vi "Browse for XNET Database.vi"(8 "error in (no error)":errorcluster) -> (0 "error out":errorcluster, 1 "J1939 Monitor Settings":T1 {"Name" format="%.0x"}, 2 "Cancel Out":bool, 3 "J1939 XNET Settings":T2={"Database"="", "Cluster"="", "Port"="", "Baud rate [Bd]"=0, "Termination"=0, "Incoming Rate"=0, "Outcoming Rate"=0, "Write Decimation"=1} {"Termination" items=["Off", "On"]})   [LabVIEW 2015, in "J1939 Addon System Explorer.lvlib"]
uses:
  J1939 Addon System Explorer.lvlib
  Types/XNET Port.ctl
  Shared/Types/XNET Settings.ctl
  Shared/Types/Monitor Settings.ctl
  <resource>/objmgr/xnet.rc
  Shared/J1939 Addon Shared.lvlib
panel:
  in  "Name":u64=1
  in  "Address":u8
  in  "Baud rate [Bd]":u32=500000
  in  "Select CAN Cluster":u16(ring) items=["j1939.Cluster"]
  in  "XNET CAN Port":T3 items=["CAN 1", "CAN 2", "CAN 3", "CAN 4", "CAN 5", "CAN 6", "CAN 7", "CAN 8"]
  in  "Cancel":bool
  in  "Select":bool
  in  "XNET Database":refnum<k21>
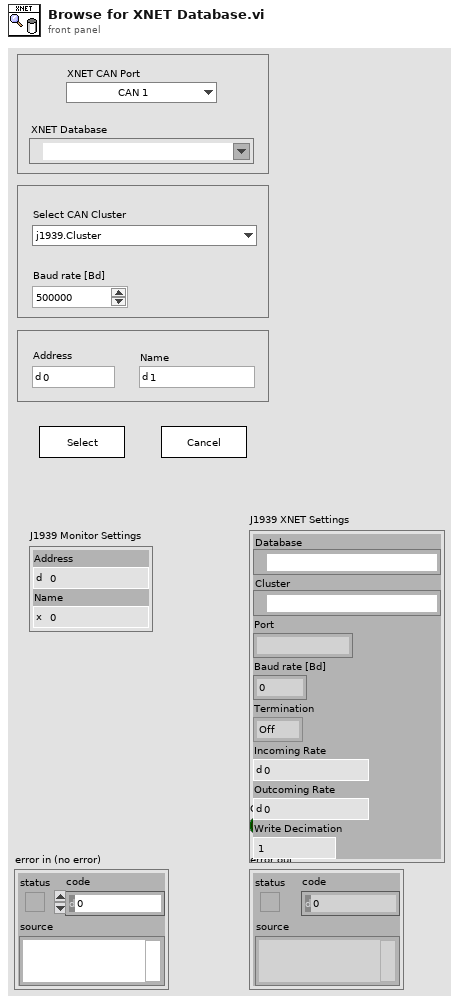
[diagram p1: front panel]
types:
  T1 = typedef "J1939 Addon Shared.lvlib/Monitor Settings.ctl" = cluster{"Address":u8, "Name":u64}
  T2 = typedef "J1939 Addon Shared.lvlib/XNET Settings.ctl" = cluster{"Database":refnum<k21>, "Cluster":refnum<k21>, "Port":string, "Baud rate [Bd]":u32, "Termination":u32, "Incoming Rate":u32, "Outcoming Rate":u32, "Write Decimation":u32}
  T3 = typedef "J1939 Addon System Explorer.lvlib/XNET Port.ctl" = u16
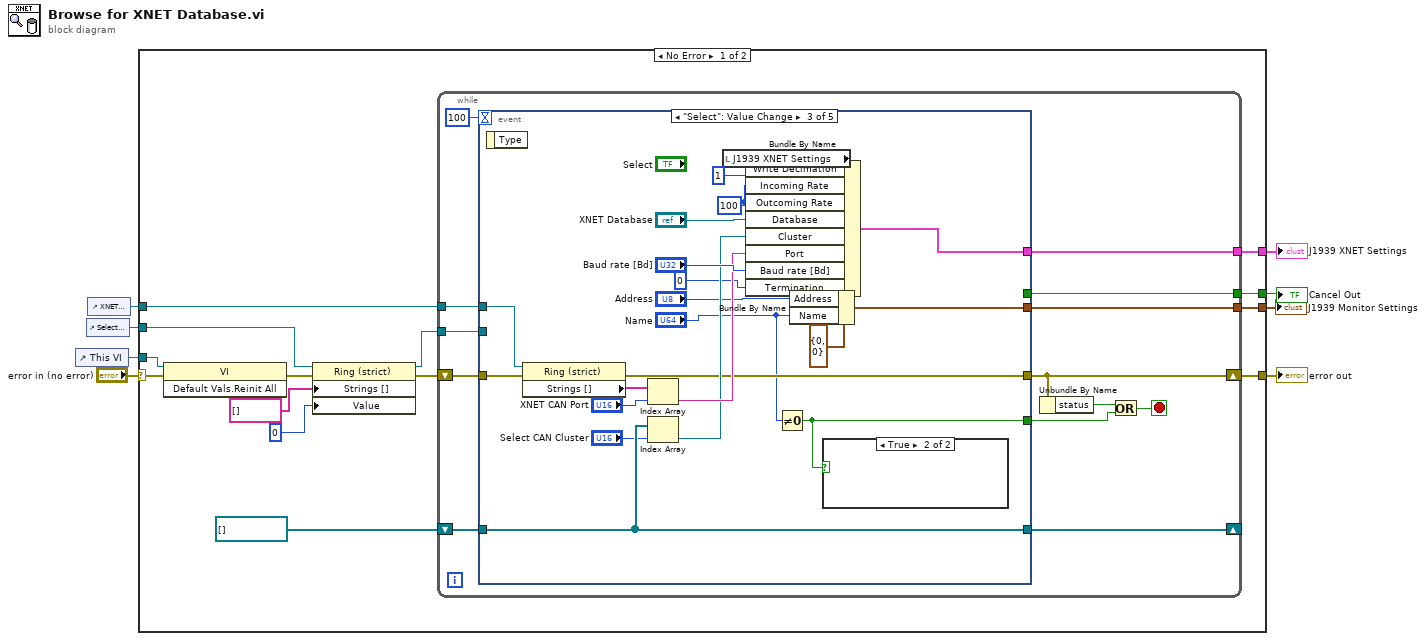
[diagram p0: block diagram]
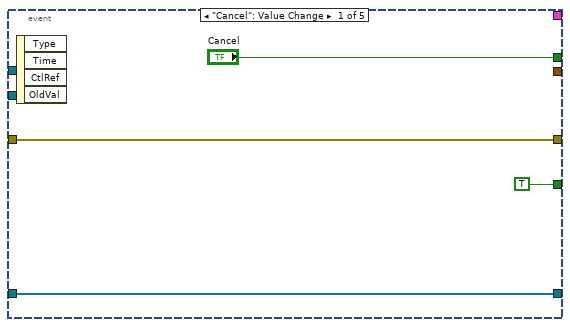
[diagram p2: hidden frame]
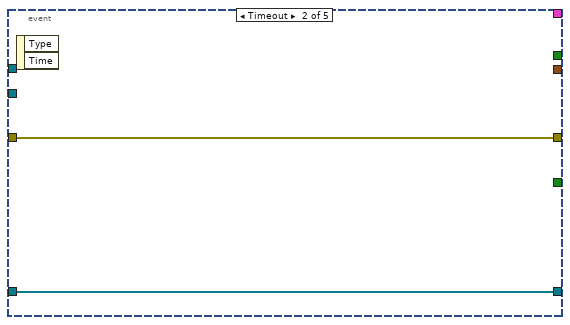
[diagram p3: hidden frame]
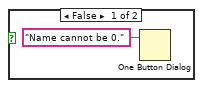
[diagram p4: hidden frame]
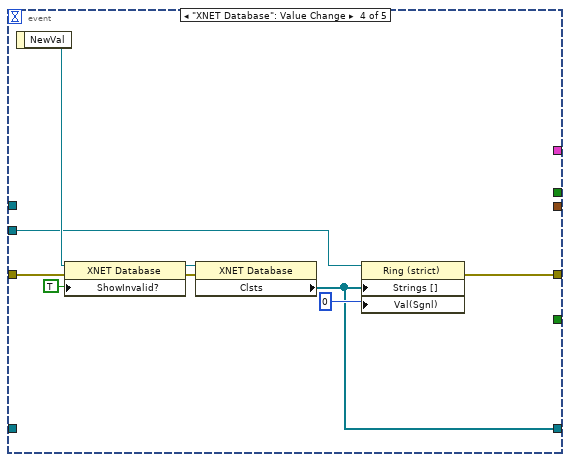
[diagram p5: hidden frame]
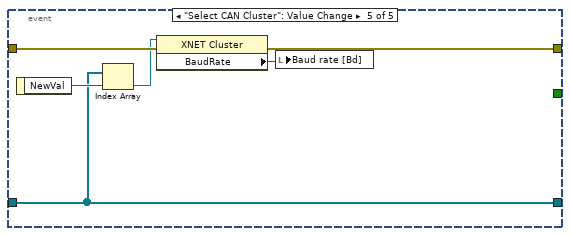
[diagram p6: hidden frame]
diagram:
  n1 = control-ref of="This VI"() -> (w5:refnum<vi>)
  n2 = control-ref of="Select CAN Cluster"() -> (w3:refnum<vi>)
  n3 = control-ref of="XNET CAN Port"() -> (w2:refnum<vi>)
  n4 = case shown="No Error" "error in (no error)" {
    selector: "error in (no error)" -> [w21 w79]
    tunnel: [w19 w79] -> w7
    tunnel: [w22 _] -> w6
    tunnel: w5 -> [w20 _]
    tunnel: [w17 _] -> w4
    tunnel: w3 -> [w16 _]
    tunnel: w2 -> [w10 _]
    tunnel: [w9 _] -> w1
    frame No Error {
      n5 = invoke class="VI" method="Default Vals.Reinit All"(reference=w20, error in=w21) -> (error out=w15:errorcluster)  [unwired: 1 in, 2 out]
      n6 = property on="Property Node" class="Ring (strict)"(reference=w16, error in=w15, "Strings []"=string[] [], "Value"=u16 0) -> (reference out=w14:refnum<vi>, error out=w13:errorcluster)
      n7 = while {
        tunnel: [w35] -> w22
        shift-right: [w33] -> _
        shift-left: refnum<k21>[] [] ("Clsts") -> [w32]
        shift-right: [w29] -> w19
        shift-left: w13 -> [w34]
        tunnel: [w31] -> w17
        tunnel: w14 -> [w25]
        tunnel: w10 -> [w24]
        tunnel: [w23] -> w9
        stop <- w26 stop-if-true
        n8 = event shown="[2] \"Select\": Value Change" {
          selector: _ -> [_ _ _ _ _]
          dyn-events: _ -> [_ _ _ _ _]
          timeout: 100 -> [_ _ _ _ _]
          tunnel: ["Cancel" _ _ _ _] -> w35
          tunnel: w34 -> [w37 w41 w53 w69 w77]
          tunnel: [w38 w40 w57 w66 w73] -> w33
          tunnel: w32 -> [w38 w40 w57 _ w73]
          tunnel: [w37 w41 w52 w64 w76] -> w29
          tunnel: [_ _ w54 _ _] -> w31
          tunnel: [TRUE _ w42 _ _] -> w27
          tunnel: w25 -> [_ _ _ w65 _]
          tunnel: w24 -> [_ _ w50 _ _]
          tunnel: [_ _ w46 _ _] -> w23
          event "Cancel": Value Change {
            n9 = event-data() -> ()  [unwired: 1 in, 4 out]
          }
          event Timeout {
            n10 = event-data() -> ()  [unwired: 1 in, 2 out]
          }
          event "Select": Value Change {
            w45 = u32 100 ("Outcoming Rate")
            n11 = event-data() -> ()  [unwired: 1 in, 1 out]
            n12 = property on="Property Node" class="Ring (strict)"(reference=w50, error in=w53) -> (error out=w52:errorcluster, "Strings []"=w51:string[])  [unwired: 1 out]
            n13 = Index Array(array=w51, index="XNET CAN Port") -> (element=w59:string)
            n14 = Index Array(array=w57, index="Select CAN Cluster") -> (element=w55:refnum<k21>)
            n15 = local read "J1939 XNET Settings"() -> (w58:T2)
            n16 = Bundle By Name(cluster=w58, "Write Decimation"=u32 1, "Incoming Rate"=w45, "Outcoming Rate"=w45, "Database"="XNET Database", "Cluster"=w55, "Port"=w59, "Baud rate [Bd]"="Baud rate [Bd]", "Termination"=u32 0) -> (w54:T2)
            n17 = Not Equal To 0?(x="Name") -> (x != 0?=w42:bool)
            n18 = Bundle By Name(cluster=T1 {"Address"=0, "Name"=0} ("J1939 Monitor Settings"), "Address"="Address", "Name"="Name") -> (w46:T1)
            n19 = case shown="True" w42 {
              frame False {
                n20 = One Button Dialog(message="Name cannot be 0.") -> ()  [unwired: 1 in, 1 out]
              }
              frame True {
              }
            }
          }
          event "XNET Database": Value Change {
            n21 = event-data() -> ("NewVal"=w68:refnum<k21>)  [unwired: 1 in]
            n22 = property class="XNET Database"(reference=w68, error in=w69, "ShowInvalid?"=TRUE ("Show Invalid From Open?")) -> (reference out=w72:refnum<k21>, error out=w71:errorcluster)
            n23 = property class="XNET Database"(reference=w72, error in=w71) -> ("Clsts"=w66:refnum<k21>[])  [unwired: 2 out]
            n24 = property on="Property Node" class="Ring (strict)"(reference=w65, "Strings []"=w66, "Val(Sgnl)"=u16 0 ("Value (Signaling)")) -> (error out=w64:errorcluster)  [unwired: 1 in, 1 out]
          }
          event "Select CAN Cluster": Value Change {
            n25 = event-data() -> ("NewVal"=w75:u16)  [unwired: 1 in]
            n26 = Index Array(array=w73, index=w75) -> (element=w74:refnum<k21>)
            n27 = property class="XNET Cluster"(reference=w74, error in=w77) -> (error out=w76:errorcluster, "BaudRate"=w78:u32)  [unwired: 1 out]
            n28 = local write "Baud rate [Bd]"(w78) -> ()
          }
        }
        n29 = Unbundle By Name(w29) -> ("status"=w28:bool)
        n30 = Or(x=w28, y=w27) -> (x .or. y?=w26:bool)
      }
    }
    frame Error {
    }
  }
  "error out" <- w7
  "Cancel Out" <- w6
  "J1939 XNET Settings" <- w4
  "J1939 Monitor Settings" <- w1
